vi "StringToNumberControl.vi"(1 "Numeric In":dbl, 2 "String In":string) -> (0 "Number Out":dbl)   [LabVIEW 2018]
doc: "Input a String and return a Number.\n\nLeave String blank, and a number returns."
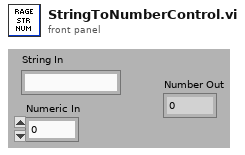
[diagram p1: front panel]
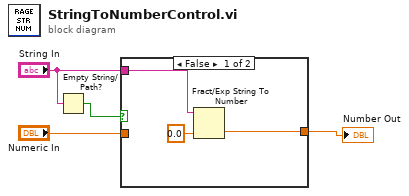
[diagram p0: block diagram]
diagram:
  n1 = Empty String/Path?(string/path="String In") -> (empty?=w2:bool)
  n2 = case shown="False" w2 {
    tunnel: [w7 w8] -> w4
    tunnel: "Numeric In" -> [_ w8]
    tunnel: "String In" -> [w6 _]
    frame False {
      n3 = Fract/Exp String To Number(string=w6, default (0 dbl)=0.0 ("default (0 DBL)")) -> (number=w7:dbl)  [unwired: 2 in, 1 out]
    }
    frame True {
    }
  }
  "Number Out" <- w4
